vi "chart series set trendline intercept.vi"(8 "error in (no error)":errorcluster, 10 "intercept":dbl, 11 "series":u32) -> (0 "error out":errorcluster, 3 "function return":u32(ring))   [LabVIEW 2015, in "xlsxwriter.lvlib"]
doc: "lxw_error chart_series_set_trendline_intercept(lxw_chart_series series, double intercept);"
uses:
  xlsxwriter.lvlib
  xlsxwriter.dll
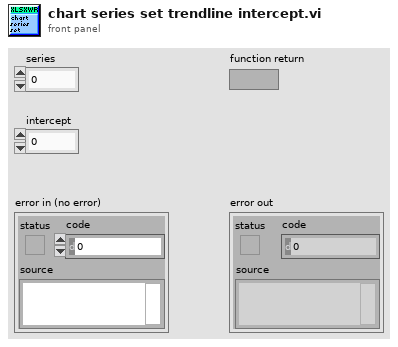
[diagram p1: front panel]
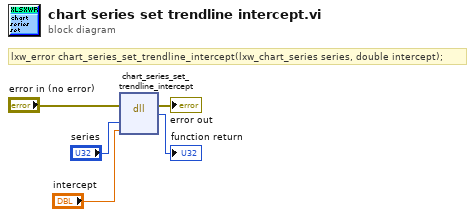
[diagram p0: block diagram]
diagram:
  # "lxw_error chart_series_set_trendline_intercept(lxw_chart_series series, double intercept);"
  n1 = dll-call lib="C:/Users/WDAGUtilityAccount/Desktop/lv_vis_added_cell/xlsxwriter.*" fn="chart_series_set_trendline_intercept"(error in="error in (no error)", "series"="series", "intercept"="intercept") -> (error out=→"error out":errorcluster, →"function return":u32)  [unwired: 4 in, 1 out]
